vi "字符串转换为数组.vi"(11 "查询内容":string) -> (3 "列首":string[](array[string]))   [LabVIEW 2013]
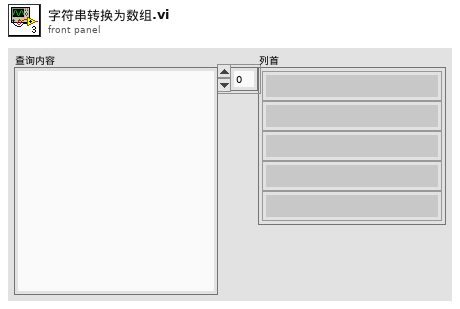
[diagram p1: front panel]
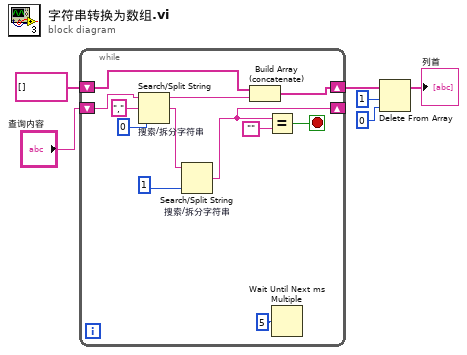
[diagram p0: block diagram]
diagram:
  n1 = while {
    shift-right: [w7] -> _
    shift-left: "查询内容" -> [w17]
    shift-right: [w15] -> w4
    shift-left: string[] [] -> [w16]
    stop <- w12 stop-if-true
    n2 = Search/Split String "搜索/拆分字符串"(string=w17, search string/char (-)="," ("搜索字符串/字符(-)"), offset (0)=0 ("偏移量(0)")) -> (substring before match=w14:string, match + rest of string=w9:string)  [unwired: 1 out]
    n3 = Search/Split String "搜索/拆分字符串"(string=w9, offset (0)=1 ("长度（剩余）")) -> (match + rest of string=w7:string)  [unwired: 1 in, 2 out]
    n4 = Build Array (concatenate)(w16, w14) -> (w15:string[])
    n5 = Equal?(x=w7, y="") -> (x = y?=w12:bool)
    n6 = Wait Until Next ms Multiple(millisecond multiple=u32 5 ("毫秒倍数")) -> ()  [unwired: 1 out]
  }
  n7 = Delete From Array(array=w4, length=1 ("长度"), index=0 ("索引")) -> (array with subset deleted=→"列首":string[])  [unwired: 1 out]
